vi "TimeCounterString.vi"(0 "date time rec":T1, 1 "negative? (F)":bool) -> (2 "String":string)   [LabVIEW 2013]
uses:
  <vilib>/Utility/miscctls.llb/LVDateTimeRec.ctl
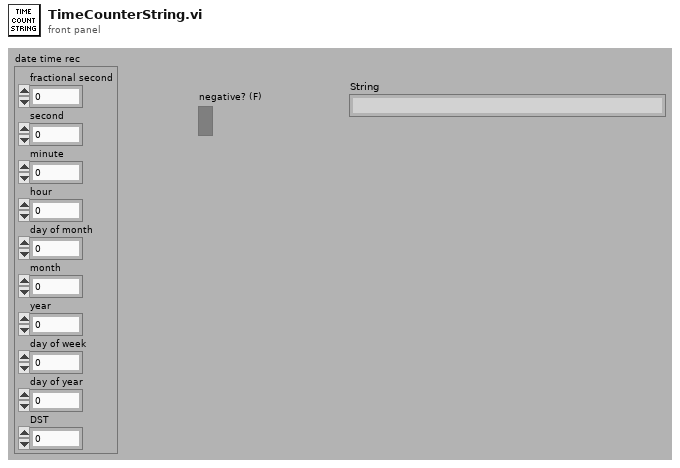
[diagram p1: front panel]
types:
  T1 = typedef "LVDateTimeRec.ctl" = cluster{"fractional second":dbl, "second":i32, "minute":i32, "hour":i32, "day of month":i32, "month":i32, "year":i32, "day of week":i32, "day of year":i32, "DST":i32}
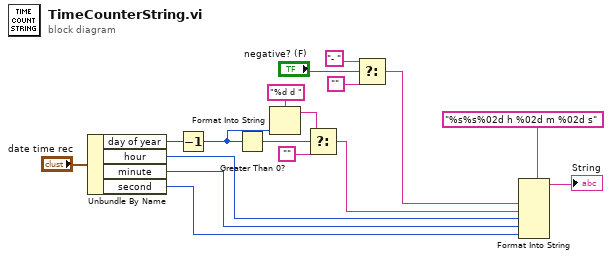
[diagram p0: block diagram]
diagram:
  n1 = Unbundle By Name("date time rec") -> ("day of year"=w17:i32, "hour"=w10:i32, "minute"=w7:i32, "second"=w6:i32)
  n2 = Decrement(x=w17) -> (x-1=w5:i32)
  n3 = Greater Than 0?(x=w5) -> (x > 0?=w13:bool)
  n4 = Format Into String(format string="%d d " ("Status"), w5) -> (resulting string=w16:string)  [unwired: 2 in, 1 out]
  n5 = Select(t=w16, s=w13, f="") -> (s? t:f=w9:string)
  n6 = Select(t="- " ("Status"), s="negative? (F)", f="") -> (s? t:f=w1:string)
  n7 = Format Into String(format string="%s%s%02d h %02d m %02d s" ("Status"), w1, w9, w10, w7, w6) -> (resulting string=→"String":string)  [unwired: 2 in, 1 out]
